vi "getArrayElementsUsingBracketedEle.vi"(8 "error in (no error)":errorcluster, 9 "requriedObject":string, 10 "brackettedElements":string, 11 "Variant in":variant) -> (0 "error out":errorcluster, 2 "error?":bool, 3 "Array Element":variant)   [LabVIEW 2015, in "Zen Analytics.lvclass"]
uses:
  Zen Analytics.lvclass
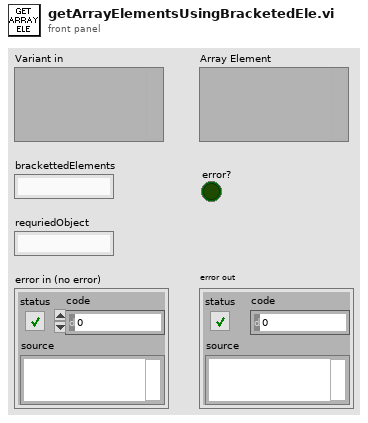
[diagram p1: front panel]
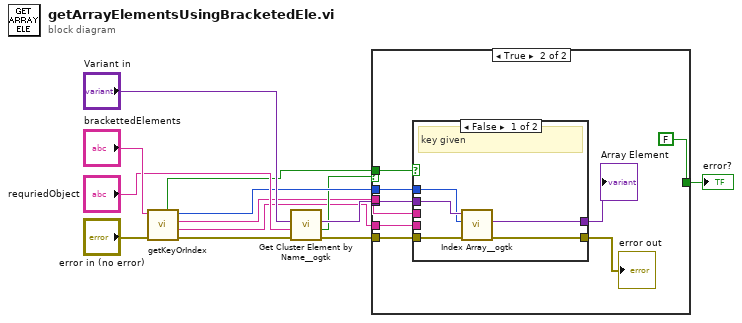
[diagram p0: block diagram]
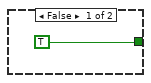
[diagram p2: hidden frame]
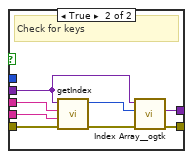
[diagram p3: hidden frame]
diagram:
  n1 = call "getKeyOrIndex.vi"("error in (no error)"="error in (no error)", "input string"="brackettedElements") -> ("error out"=w12:errorcluster, "value"=w1:string, "key"=w2:string, "index"=w6:i32, "keygiven?"=w3:bool)  [unwired: 5 in]
  n2 = call <userlib>:"Get Cluster Element by Name__ogtk.vi"("error in (no error)"=w12, "Element Name"="requriedObject", "Cluster"="Variant in") -> ("error out"=w10:errorcluster, "found?"=w4:bool, "VElement"=w8:variant)  [unwired: 6 in]
  n3 = case shown="True" w4 {
    tunnel: w3 -> [_ w23]
    tunnel: w10 -> [_ w22]
    tunnel: w8 -> [_ w21]
    tunnel: w1 -> [_ w20]
    tunnel: w2 -> [_ w19]
    tunnel: w6 -> [_ w18]
    tunnel: [TRUE FALSE] -> w5
    frame False {
    }
    frame True {
      n4 = case shown="False" w23 {
        tunnel: [w28 w29] -> w16
        tunnel: [w27 w30] -> w17
        tunnel: w21 -> [w26 w32]
        tunnel: w22 -> [w25 w35]
        tunnel: w18 -> [w24 _]
        tunnel: w19 -> [_ w36]
        tunnel: w20 -> [_ w34]
        frame False {
          # "key given"
          n5 = call <userlib>:"Index Array__ogtk.vi"("error in (no error)"=w25, "Index (1D)"=w24, "MultiD Array"=w26) -> ("error out"=w27:errorcluster, "Array Element"=w28:variant)  [unwired: 7 in]
        }
        frame True {
          # "Check for keys"
          n6 = call "getIndex.vi"("error in (no error)"=w35, "value"=w34, "key"=w36, "VElement"=w32) -> ("error out"=w31:errorcluster, "indexOut"=w33:i32)  [unwired: 6 in]
          n7 = call <userlib>:"Index Array__ogtk.vi"("error in (no error)"=w31, "Index (1D)"=w33, "MultiD Array"=w32) -> ("error out"=w30:errorcluster, "Array Element"=w29:variant)  [unwired: 7 in]
        }
      }
      "error out" <- w17
      "Array Element" <- w16
    }
  }
  "error?" <- w5
